vi "KeyenceCVX.Main-Scan.Product.vi"(8 "error in":errorcluster, 9 "Code sets in":T4={"Ready"=FALSE, "DoubleOrder"=FALSE, "OrderDone"=FALSE, "AllowSingleSlot"=FALSE, "IgnoreOCR"=FALSE, "ThresholdA"=0, "ThresholdB"=0, "Plate"=enum."Wabco", "ImgPath"=path "", "Variant"={"State"=enum."Init", "ImgPath"=path "", "WabcoPlate"="", "WabcoProduct"="", "ClientProduct"="", "ClientPlate"="", "TotalQuantity"=0, "OrderQuantity"=0, "Serial"=0, "Wabco"={"LaserJob"="", "AdditionalTxt"="037", "FactoryCode"="", "RevID"=0, "ForkID"=0, "FailuresLimit"=0, "GlobalCnt"=0, "ScannerProgram"=0, "SerialFormat"=enum."6 dig", "CoordA"={"X"=0.0, "Y"=0.0, "Angle"=0.0}, "CoordB"={"X"=0.0, "Y"=0.0, "Angle"=0.0}, "DMCconfig"=0, "CVX_Program"=0}, "Client"={"LaserJob"="", "AdditionalTxt"="", "FactoryCode"="037", "RevID"=0, "ForkID"=0, "FailuresLimit"=0, "GlobalCnt"=0, "ScannerProgram"=0, "SerialFormat"=enum."6 dig", "CoordA"={"X"=0.0, "Y"=0.0, "Angle"=0.0}, "CoordB"={"X"=0.0, "Y"=0.0, "Angle"=0.0}, "DMCconfig"=0, "CVX_Program"=0}}}, 10 "CodeB":T1, 11 "CodeA":T1) -> (0 "error out":errorcluster, 2 "CodeB out":T1, 3 "CodeA out":T1)   [LabVIEW 2016]
uses:
  Sequence/Sequence.Code.Sets.ctl
  Sequence/Sequence.PlateType.ctl
  Logger/Logger.Variant.Sets.ctl
  Station/Station.Changeover.State.vi
  Station/Station.Plate.Properties.ctl
  Sequence/Sequence.Code.SerialFormat.ctl
  V7310/LowLevel/V7310.Job.Sets.ctl
  Sequence/Sequence.Prod.StatusData.ctl
  Sequence/Sequence.Step.Status.ctl
  Sequence/Sequence.Test.BreakReason.ctl
  private/controls/TriggerNo.ctl
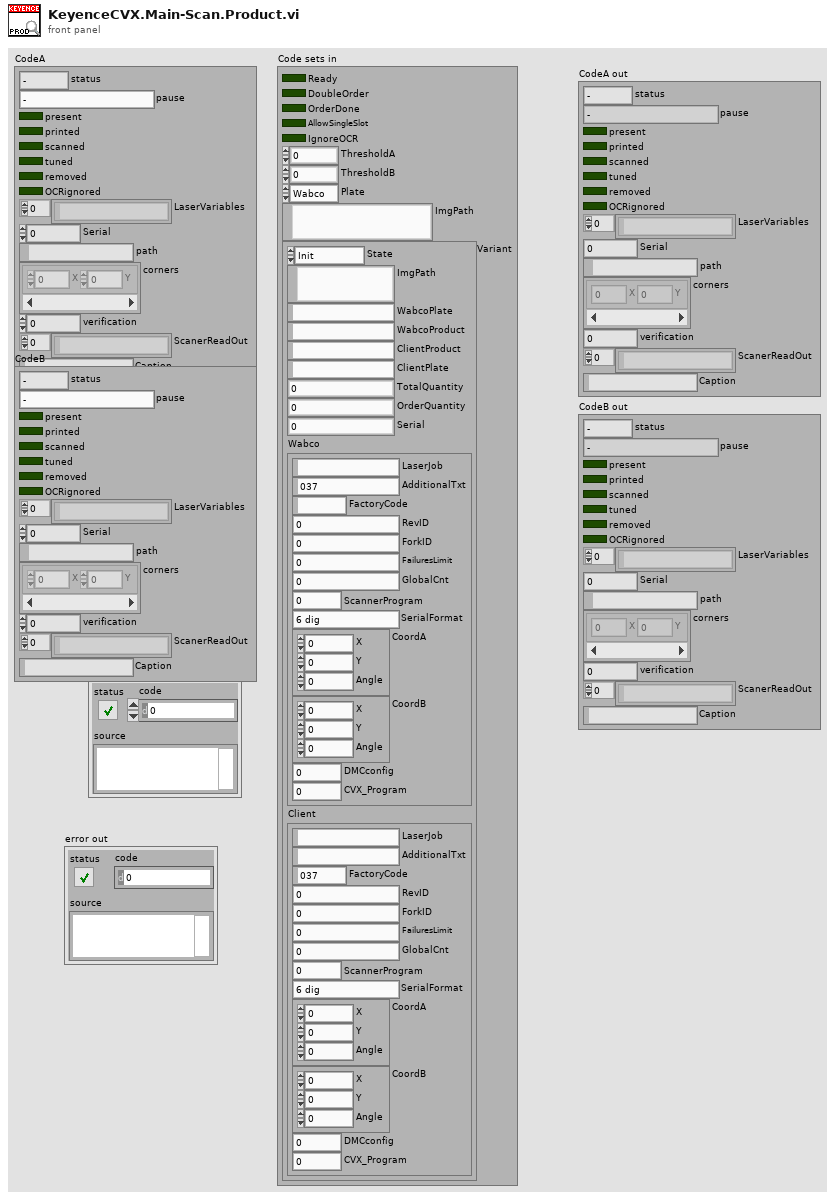
[diagram p1: front panel]
types:
  T1 = typedef "Sequence.Prod.StatusData.ctl" = cluster{"status":T2, "pause":T3, "present":bool, "printed":bool, "scanned":bool, "tuned":bool, "removed":bool, "OCRignored":bool, "LaserVariables":string[], "Serial":i32, "path":path, "corners":cluster{"X":i32, "Y":i32}[], "verification":u8, "ScanerReadOut":string[], "Caption":string}
  T2 = typedef "Sequence.Step.Status.ctl" = enum16{"-", "Pending", "Running", "Skipped", "Passed", "Failed", "Done", "Error", "Aborted", "Stopped"}
  T3 = typedef "Sequence.Test.BreakReason.ctl" = enum16{"-", "NOK container", "OK container", "Rev empty", "Rev missing", "Rev wrong", "Fork missing", "Fork wrong", "NOK limit", "Unload failure", "Single slot", "Part done", "Err: Prod move work", "Err: Prod move home", "Err: Prod lift work", "Err: Prod lift home", "Err: Prod Arm Work", "Err: Prod Arm NOK", "Err: Prod Arm OK", "Err: Prod NOK suck", "Err: Prod NOK drop", "Err: Prod OK missing", "Err: Prod OK suck", "Err: Prod OK drop"}
  T4 = typedef "Sequence.Code.Sets.ctl" = cluster{"Ready":bool, "DoubleOrder":bool, "OrderDone":bool, "AllowSingleSlot":bool, "IgnoreOCR":bool, "ThresholdA":u8, "ThresholdB":u8, "Plate":T5, "ImgPath":path, "Variant":T6}
  T5 = typedef "Sequence.PlateType.ctl" = enum16{"Wabco", "Client"}
  T6 = typedef "Logger.Variant.Sets.ctl" = cluster{"State":T7, "ImgPath":path, "WabcoPlate":string, "WabcoProduct":string, "ClientProduct":string, "ClientPlate":string, "TotalQuantity":u16, "OrderQuantity":u16, "Serial":i32, "Wabco":T8, "Client":T8}
  T7 = typedef "Station.Changeover.State.vi" = enum16{"Init", "Scaning", "NOK", "Wait for ack", "Ready"}
  T8 = typedef "Station.Plate.Properties.ctl" = cluster{"LaserJob":string, "AdditionalTxt":string, "FactoryCode":string, "RevID":u8, "ForkID":u8, "FailuresLimit":u16, "GlobalCnt":i32, "ScannerProgram":u8, "SerialFormat":T9, "CoordA":T10, "CoordB":T10, "DMCconfig":i32, "CVX_Program":u16}
  T9 = typedef "Sequence.Code.SerialFormat.ctl" = enum8{"", "6 dig", "7 dig"}
  T10 = typedef "V7310.Job.Sets.ctl" = cluster{"X":dbl, "Y":dbl, "Angle":dbl}
  T11 = typedef "TriggerNo.ctl" = u8
  T12 = typedef "KeyenceCVX.CodeDetails.ctl" = cluster{"text":string, "status":bool, "ImgPathA":path, "ImgPathB":path}
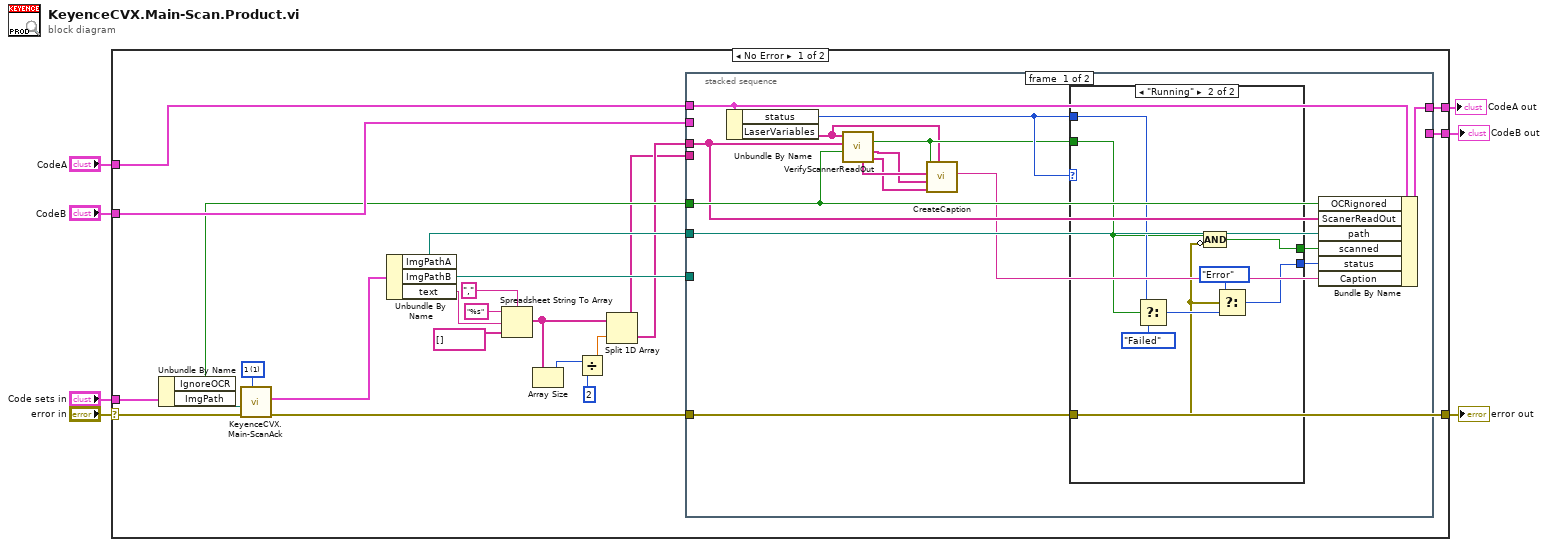
[diagram p0: block diagram]
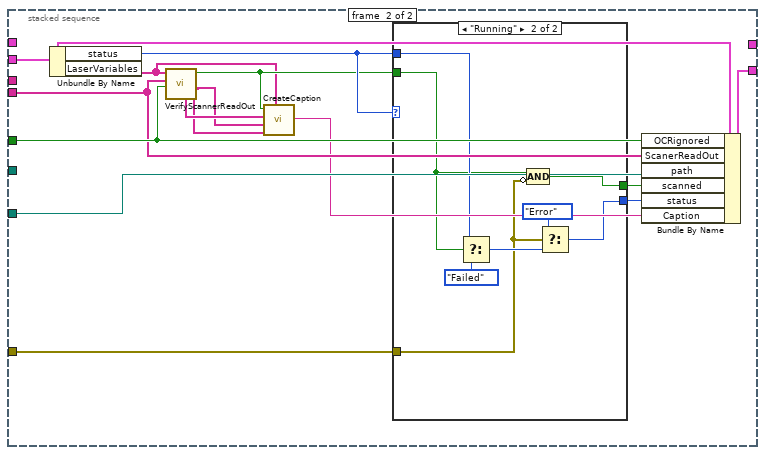
[diagram p3: hidden frame]
diagram:
  n1 = case shown="No Error" "error in" {
    selector: "error in" -> [w30 w81]
    tunnel: [w22 w81] -> w6
    tunnel: "Code sets in" -> [w28 _]
    tunnel: "CodeA" -> [w27 w80]
    tunnel: [w29 w80] -> w3
    tunnel: "CodeB" -> [w20 w79]
    tunnel: [w19 w79] -> w1
    frame No Error {
      w18 = T11 1 items=["1"=1, "2"=2, "3"=3, "4"=4, "ALL"=5] ("TriggerNo")
      n2 = Unbundle By Name(w28) -> ("IgnoreOCR"=w16:bool, "ImgPath"=w17:path)
      n3 = call "KeyenceCVX.Main-ScanAck.vi"("TriggerNo"=w18, "error in"=w30, "imgpath"=w17) -> ("error out"=w22:errorcluster, "CVX Readout details"=w21:T12)  [unwired: 6 in, 1 out]
      n4 = Unbundle By Name(w21) -> ("ImgPathA"=w14:path, "ImgPathB"=w13:path, "text"=w26:string)
      n5 = Spreadsheet String To Array(delimiter (Tab)=",", format string="%s", spreadsheet string=w26, array type (2D Dbl)=string[] []) -> (array=w15:string[])
      n6 = Array Size(array=w15) -> (size(s)=w10:i32)
      n7 = Divide(x=w10, y=2) -> (x/y=w11:dbl)
      n8 = Split 1D Array(array=w15, index=w11) -> (first subarray=w8:string[], second subarray=w9:string[])
      n9 = stacked-sequence {
        tunnel: w14 -> [w45 _]
        tunnel: [w44 _] -> w29
        tunnel: w27 -> [w40 _]
        tunnel: w9 -> [w37 _]
        tunnel: w22 -> [w41 w67]
        tunnel: w20 -> [_ w65]
        tunnel: [_ w64] -> w19
        tunnel: w8 -> [_ w61]
        tunnel: w16 -> [w38 w63]
        tunnel: w13 -> [_ w62]
        frame #0 {
          n10 = Unbundle By Name(w40) -> ("status"=w39:T2, "LaserVariables"=w35:string[])
          n11 = call "VerifyScannerReadOut.vi"("IgnoreOCR"=w38, "ScanerReadOut"=w37, "LaserVariables"=w35) -> ("WrongScannerRead"=w32:string[], "WrongLaserVar"=w33:string[], "Equal"=w36:bool, "WrongVarName"=w34:string[])  [unwired: 4 in, 1 out]
          n12 = call "CreateCaption.vi"("LaserVariables"=w35, "WrongScannerRead"=w32, "WrongLaserVar"=w33, "WrongVarName"=w34, "Equal"=w36) -> ("Caption"=w31:string)  [unwired: 6 in]
          n13 = case shown="\"Running\"" w39 {
            tunnel: w41 -> [_ w49]
            tunnel: w36 -> [_ w47]
            tunnel: [_ w48] -> w43
            tunnel: [w46 w52] -> w42
            tunnel: w39 -> [w46 w50]
            frame Default {
            }
            frame "Running" {
              n14 = Select(t=w50, s=w47, f=Sequence.Step.Status."Failed" ("status")) -> (s? t:f=w51:T2)
              n15 = Compound Arithmetic op=AND(w47, invert w49) -> (w48:bool)
              n16 = Select(t=Sequence.Step.Status."Error" ("status"), s=w49, f=w51) -> (s? t:f=w52:T2)
            }
          }
          n17 = Bundle By Name(cluster=w40, "OCRignored"=w38, "ScanerReadOut"=w37, "path"=w45, "scanned"=w43, "status"=w42, "Caption"=w31) -> (w44:T1)
        }
        frame #1 {
          n18 = Unbundle By Name(w65) -> ("status"=w66:T2, "LaserVariables"=w59:string[])
          n19 = call "VerifyScannerReadOut.vi"("IgnoreOCR"=w63, "ScanerReadOut"=w61, "LaserVariables"=w59) -> ("WrongScannerRead"=w56:string[], "WrongLaserVar"=w57:string[], "Equal"=w60:bool, "WrongVarName"=w58:string[])  [unwired: 4 in, 1 out]
          n20 = call "CreateCaption.vi"("LaserVariables"=w59, "WrongScannerRead"=w56, "WrongLaserVar"=w57, "WrongVarName"=w58, "Equal"=w60) -> ("Caption"=w55:string)  [unwired: 6 in]
          n21 = case shown="\"Running\"" w66 {
            tunnel: w67 -> [_ w73]
            tunnel: w60 -> [_ w71]
            tunnel: [_ w72] -> w69
            tunnel: [w70 w76] -> w68
            tunnel: w66 -> [w70 w74]
            frame Default {
            }
            frame "Running" {
              n22 = Select(t=w74, s=w71, f=Sequence.Step.Status."Failed" ("status")) -> (s? t:f=w75:T2)
              n23 = Compound Arithmetic op=AND(w71, invert w73) -> (w72:bool)
              n24 = Select(t=Sequence.Step.Status."Error" ("status"), s=w73, f=w75) -> (s? t:f=w76:T2)
            }
          }
          n25 = Bundle By Name(cluster=w65, "OCRignored"=w63, "ScanerReadOut"=w61, "path"=w62, "scanned"=w69, "status"=w68, "Caption"=w55) -> (w64:T1)
        }
      }
    }
    frame Error {
    }
  }
  "error out" <- w6
  "CodeA out" <- w3
  "CodeB out" <- w1
